vi "USRP Stream to Disk Queues USRP and Binary File IO.vi"() -> ()   [LabVIEW 2016]
doc: "Recommended Input Signal: 100 MHz, 0dBm, sine wave\n\nThis example requires NI-RFSA 2.0.1 or later.\nDevices Supported: NI PXI-5661\n\nVI Description:\nThis example demonstrates using continuous acquisition to fetch IQ data while continuously streaming the data to a binary file using the Win32 File I/O VIs. The vertical range and the IQ rate of the NI Vector Signal Analyzer (VSA) are configured using the NI-RFSA VIs. The VSA is configured to run continuously with the niRFSA Configure Number of Samples.vi, and data is continuously fetched from the onboard memory of the device within the producer loop using the niRFSA Fetch IQ.vi.\n\nThe producer loop continuously fetches data from onboard memory into the LabVIEW memory using DMA transfers. This data is placed into a queue in order to efficiently transfer the data to a parallel consumer loop where it is written file. If the sampling rate is low, the computer can fetch all the data from the VSA, so data is never overwritten. However, at faster sampling rates, the computer will not be able to fetch the data before it is overwritten by new data. This results in the \"data overwritten\" error.\n\nThe consumer loop continuously empties data from the queue and writes data to disk using the Win32 Write File.vi. The file is opened using the Win32 Open File.vi, which disables Windows caching during the write process, resulting in increased performance. However when Windows caching is disabled, <b>data must be written to file in a multiple of the sector size of the disk (typically 512 bytes).</b>"
uses:
  <instrlib>/niUSRP/niUSRP Fetch Rx Data (I16).vi
panel:
  out "error out":errorcluster
  in  "active antenna":string
  in  "device names":refnum<k15>
  out "Elements in Queue":i32(slide) scale=0.0..8.0 scale format="%0.0f"
  in  "Max Queue Size":i32=8
  in  "error in":errorcluster {"code" format="%.0x"}
  in  "reference level (dBm)":dbl format="%.2f"
  in  "IQ rate (S/s)":dbl=25000000.0 format="%#_6p"
  in  "carrier frequency":dbl=100000000.0 format="%#_6p"
  in  "Samples Per Fetch":i64=4194304 caption="Max Points Per Fetch" step=1048576
  out "ErrorInConsumer":bool=TRUE
  in  "stop":bool
  out "Acquisition Status":bool
  out "Total Samples Fetched":u64 format="%.3p"
  in  "Total Samples to Acquire":u64=10000269312 step=1048576 format="%.3p"
  in  "Destination File":path=path "C:/BinaryIQData.bin"
  # "Acquire IQ Data and Write to Disk Using Binary File I/O VIs"
  # "Buffer and File Configuration"
  # "USRP Configuration"
  # "(should be a multiple of disk sector size)"
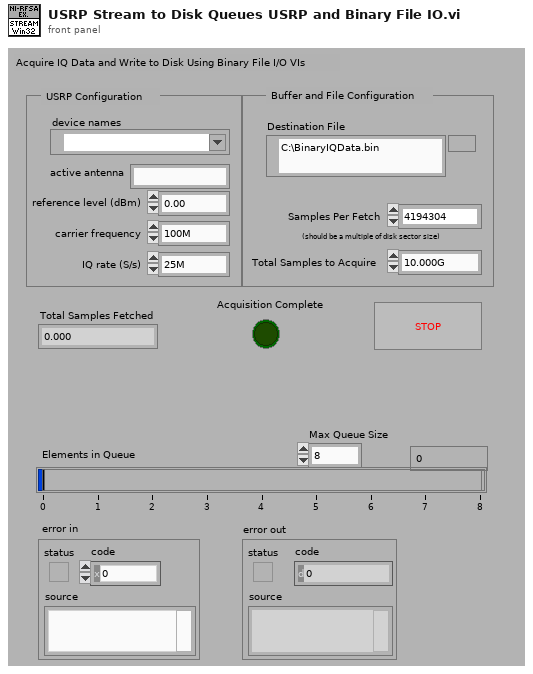
[diagram p1: front panel]
types:
  T1 = enum16{"open", "replace", "create", "open or create", "replace or create", "replace or create with confirmation"}
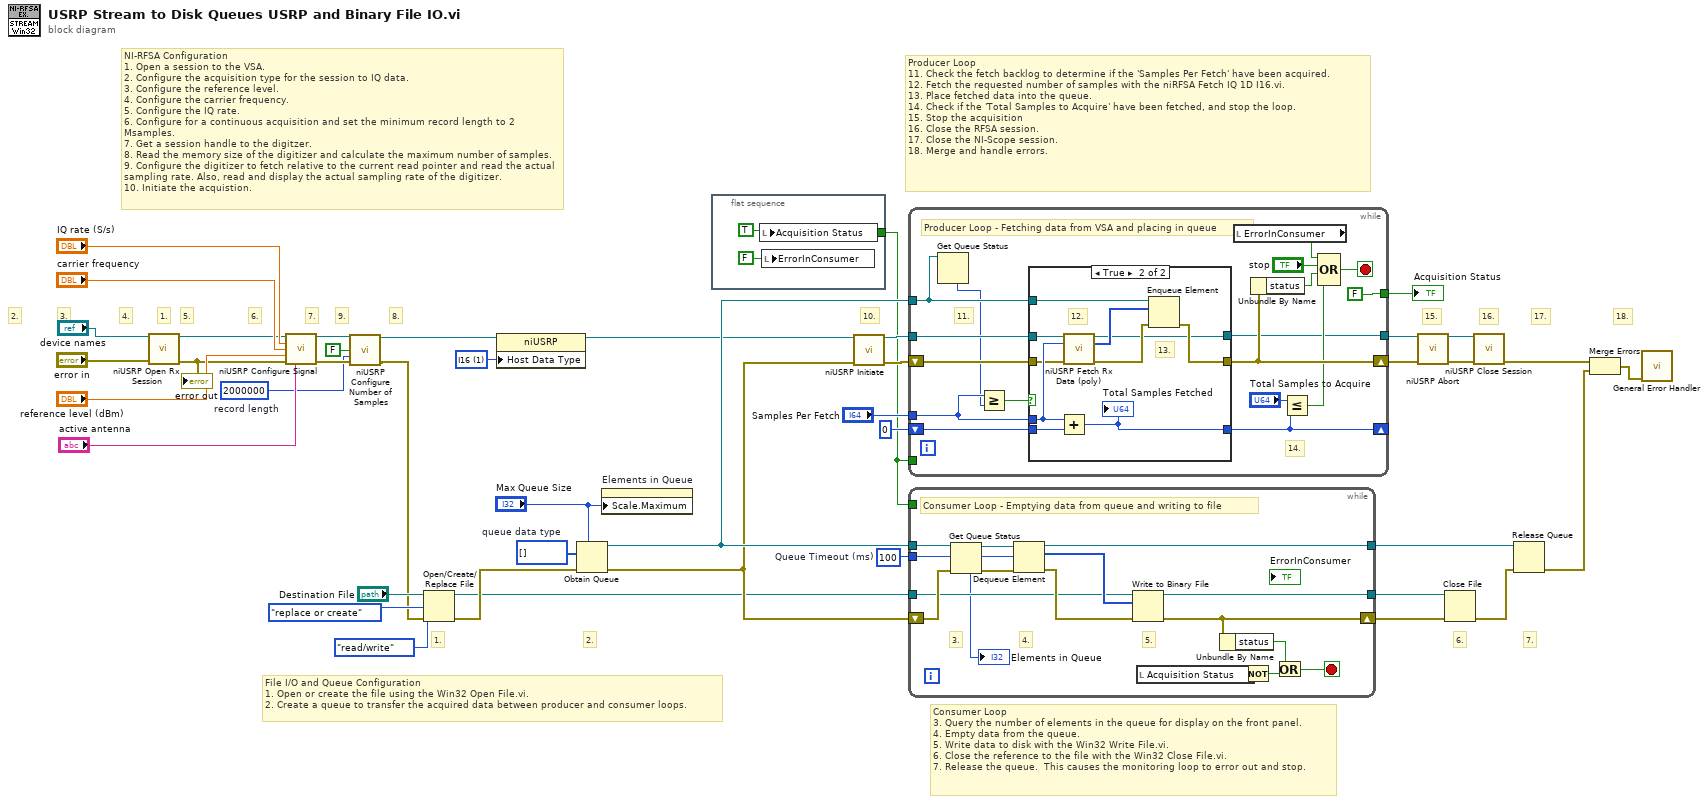
[diagram p0: block diagram]
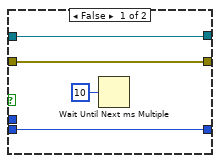
[diagram p2: hidden frame]
diagram:
  w1 = 1 items=["CDB", "I16"] ("Configuration:Advanced:Host Data Type")
  w40 = i16[] []  # queue data type
  w41 = 100  # Queue Timeout (ms)
  w5 = 2000000  # record length
  # "7."
  # "6."
  # "Consumer Loop\n3. Query the number of elements in the queue for display on the front panel.\n4. Empty data from the queue.\n5. Write data to disk with the Win32 Write File.vi.\n6. Close the reference to the file with the Win32 Close File.vi.\n7. Release the queue.  This causes the monitoring loop to error out and stop."
  # "18."
  # "17."
  # "16."
  # "15."
  # "Producer Loop\n11. Check the fetch backlog to determine if the 'Samples Per Fetch' have been acquired.\n12. Fetch the requested number of samples with the niRFSA Fetch IQ 1D I16.vi.\n13. Place fetched data into the queue.\n14. Check if the 'Total Samples to Acquire' have been fetched, and stop the loop.\n15. Stop the acquisition\n16. Close the RFSA session.\n17. Close the NI-Scope session.\n18. Merge and handle errors."
  # "2."
  # "1."
  # "File I/O and Queue Configuration\n1. Open or create the file using the Win32 Open File.vi.\n2. Create a queue to transfer the acquired data between producer and consumer loops."
  # "10."
  # "9."
  # "8."
  # "7."
  # "6."
  # "5."
  # "4."
  # "3."
  # "2."
  # "1."
  # "NI-RFSA Configuration\n1. Open a session to the VSA.\n2. Configure the acquisition type for the session to IQ data.\n3. Configure the reference level.\n4. Configure the carrier frequency.\n5. Configure the IQ rate.\n6. Configure for a continuous acquisition and set the minimum record length to 2 Msamples.\n7. Get a session handle to the digitzer.\n8. Read the memory size of the digitizer and calculate the maximum number of samples.\n9. Configure the digitizer to fetch relative to the current read pointer and read the actual sampling rate. Also, read and display the actual sampling rate of the digitizer.\n10. Initiate the acquistion."
  n1 = call <instrlib>:"niUSRP Open Rx Session.vi"("device names"="device names", "error in (no error)"="error in") -> ("session handle out"=w11:refnum<k15>, "error out"=w12:errorcluster)  [unwired: 12 in]
  "error out" <- w12
  n2 = call <instrlib>:"niUSRP Configure Signal.vi"("session handle"=w11, "IQ rate"="IQ rate (S/s)", "carrier frequency"="carrier frequency", "gain"="reference level (dBm)", "error in (no error)"=w12, "active antenna"="active antenna") -> ("session handle out"=w6:refnum<k15>, "error out"=w7:errorcluster)  [unwired: 5 in, 3 out]
  n3 = call <instrlib>:"niUSRP Configure Number of Samples.vi"("session handle"=w6, "number of samples is finite"=FALSE, "number of samples"=w5, "error in (no error)"=w7) -> ("session handle out"=w3:refnum<k15>, "error out"=w8:errorcluster)  [unwired: 10 in]
  n4 = Open/Create/Replace File(file path (use dialog)="Destination File", error in=w8, operation (0:open)=T1."replace or create", access (0:read/write)=enum16{"read/write", "read-only", "write-only"}."read/write") -> (refnum out=w20:refnum<file>, error out=w38:errorcluster)  [unwired: 2 in, 1 out]
  n5 = property class="niUSRP"(reference=w3, "Host Data Type"=w1) -> (reference out=w2:refnum<k15>)  [unwired: 1 in, 1 out]
  n6 = Obtain Queue(max queue size (-1, unlimited)="Max Queue Size", element data type=w40, error in (no error)=w38) -> (queue out=w36:refnum<queue>, error out=w33:errorcluster)  [unwired: 2 in, 1 out]
  n7 = property on="Elements in Queue" class="Slide (strict)"("Scale.Maximum"="Max Queue Size") -> ()  [unwired: 2 in, 2 out]
  n8 = flat-sequence {
    tunnel: [w44] -> w26
    frame #0 {
      w44 = TRUE ("Acquisition Done")
      n9 = local write "Acquisition Status"(w44) -> ()
      n10 = local write "ErrorInConsumer"(FALSE ("Acquisition Done")) -> ()
    }
  }
  n11 = call <instrlib>:"niUSRP Initiate.vi"("session handle"=w2, "error in (no error)"=w33) -> ("session handle out"=w34:refnum<k15>, "error out"=w32:errorcluster)  [unwired: 12 in]
  n12 = while {
    shift-right: [w51] -> _
    shift-left: u64 0 ("Samples to Take") -> [w52]
    tunnel: [FALSE ("Acquisition Done")] -> w42
    tunnel: w36 -> [w47]
    shift-right: [w61] -> w30
    shift-left: w32 -> [w48]
    tunnel: "Samples Per Fetch" -> [w53]
    tunnel: w34 -> [w49]
    tunnel: [w50] -> w17
    tunnel: w26 -> [_]
    stop <- w57 stop-if-true
    # "14."
    # "11."
    # "Producer Loop - Fetching data from VSA and placing in queue"
    n13 = Get Queue Status(queue=w47) -> (# elements in queue=w46:i32)  [unwired: 2 in, 7 out]
    n14 = Greater Or Equal?(x=w53, y=w46) -> (x >= y?=w54:bool)
    n15 = case shown="True" w54 {
      tunnel: [w66 w73] -> w61
      tunnel: w47 -> [_ w74]
      tunnel: w48 -> [w66 w71]
      tunnel: w53 -> [_ w72]
      tunnel: w52 -> [w65 w76]
      tunnel: [w65 w75] -> w51
      tunnel: w49 -> [w63 w67]
      tunnel: [w63 w68] -> w50
      frame False {
        n16 = Wait Until Next ms Multiple(millisecond multiple=u32 10 ("milliseconds to wait")) -> ()  [unwired: 1 out]
      }
      frame True {
        # "13."
        # "12."
        n17 = Add(x=w72, y=w76) -> (x+y=w75:u64)
        "Total Samples Fetched" <- w75
        n18 = call-poly <instrlib>:"niUSRP Fetch Rx Data (poly).vi"("session handle"=w67, "number of samples"=w72, "error in (no error)"=w71) -> ("session handle out"=w68:refnum<k15>, "data"=w69:i16[], "error out"=w70:errorcluster)  [unwired: 9 in, 1 out]
        n19 = Enqueue Element(queue=w74, element=w69, error in (no error)=w70) -> (error out=w73:errorcluster)  [unwired: 1 in, 2 out]
      }
    }
    n20 = local read "ErrorInConsumer"() -> (w60:bool)
    n21 = Unbundle By Name(w61) -> ("status"=w58:bool)
    n22 = Less Or Equal?(x="Total Samples to Acquire", y=w51) -> (x <= y?=w55:bool)
    n23 = Compound Arithmetic op=OR(w60, "stop", w58, w55) -> (w57:bool)
  }
  "Acquisition Status" <- w42
  n24 = while {
    tunnel: w41 -> [w92]
    tunnel: w36 -> [w87]
    shift-right: [w79] -> w23
    shift-left: w33 -> [w85]
    tunnel: [w88] -> w37
    tunnel: w26 -> [_]
    tunnel: [w82] -> w22
    tunnel: w20 -> [w80]
    stop <- w90 stop-if-true
    # "5."
    # "4."
    # "3."
    # "Consumer Loop - Emptying data from queue and writing to file"
    n25 = Get Queue Status(queue=w87, error in (no error)=w85) -> (queue out=w86:refnum<queue>, error out=w84:errorcluster, # elements in queue=→"Elements in Queue":i32)  [unwired: 1 in, 5 out]
    n26 = Dequeue Element(queue=w86, timeout in ms (-1)=w92, error in (no error)=w84) -> (queue out=w88:refnum<queue>, element=w83:i16[], error out=w81:errorcluster)  [unwired: 1 out]
    n27 = Write to Binary File(file (use dialog)=w80, data=w83, error in=w81) -> (refnum out=w82:refnum<file>, error out=w79:errorcluster)  [unwired: 3 in, 1 out]
    n28 = local read "Acquisition Status"() -> (w91:bool)
    n29 = Unbundle By Name(w79) -> ("status"=w78:bool)
    n30 = Not(x=w91) -> (.not. x?=w89:bool)
    n31 = Or(x=w78, y=w89) -> (x .or. y?=w90:bool)
  }
  n32 = call <instrlib>:"niUSRP Abort.vi"("session handle"=w17, "error in (no error)"=w30) -> ("session handle out"=w28:refnum<k15>, "error out"=w29:errorcluster)  [unwired: 12 in]
  n33 = Close File(refnum=w22, error in=w23) -> (error out=w24:errorcluster)  [unwired: 1 out]
  n34 = call <instrlib>:"niUSRP Close Session.vi"("session handle"=w28, "error in (no error)"=w29) -> ("error out"=w16:errorcluster)  [unwired: 13 in]
  n35 = Release Queue(queue=w37, error in (no error)=w24) -> (error out=w31:errorcluster)  [unwired: 1 in, 2 out]
  n36 = Merge Errors(w16, w31) -> (w25:errorcluster)
  n37 = call <vilib>:"General Error Handler.vi"("error in (no error)"=w25) -> ()  [unwired: 10 in, 5 out]
